vi "RegisterReader.vi"(7 "error in (no error)":errorcluster, 10 "connection ID":refnum<k5>) -> (0 "error out":errorcluster, 3 "connection ID out":refnum<k5>)   [LabVIEW 2009]
panel:
  in  "Register Number":u16=4
  out "Register Read":dbl[](array[numeric])
  out "Register read":u32
  in  "Device":u16(ring)=4 items=["Attenuation", "Clipping", "Enable channel", "Delay line", "ASIC"]
  # "0     1     2     3     4    5     6     7     8    9    10   11  12   13   14   15"
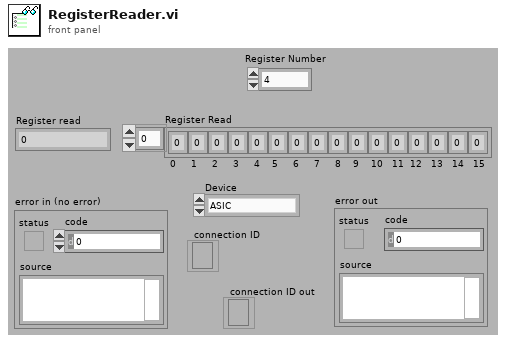
[diagram p1: front panel]
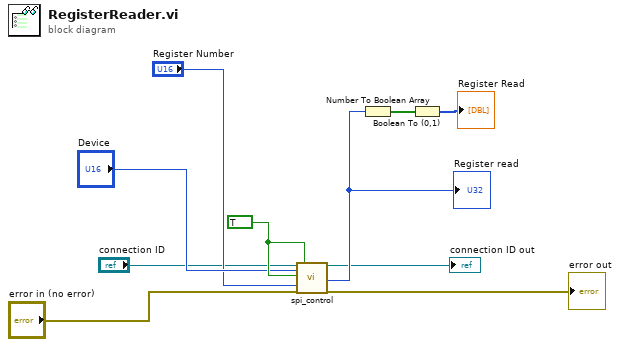
[diagram p0: block diagram]
diagram:
  w8 = TRUE
  n1 = call "spi_control.vi"("connection ID"="connection ID", "Device"="Device", "Read/#write"=w8, "Register or channel"="Register Number", "error out 3"="error in (no error)", "Read physical"=w8) -> ("connection ID out"=→"connection ID out":refnum<k5>, "data read value"=w7:u32, "error out 2"=→"error out":errorcluster)  [unwired: 6 in, 5 out]
  "Register read" <- w7
  n2 = Number To Boolean Array(number=w7) -> (Boolean array=w9:bool[])
  n3 = Boolean To (0,1)(Boolean=w9) -> (0, 1=→"Register Read":i16[])
